vi "VIQueryBuildSpecs.vi"(8 "Error In":errorcluster, 11 "Project Path":string) -> (0 "Error Out":errorcluster, 3 "Targets":T1[](array[typedef]))   [LabVIEW 2013]
uses:
  VIProject/VPTargetBuildSpecs.ctl
  VIProject/VPBuildSpecInformation.ctl
  VIProject/VIProject.lvlib
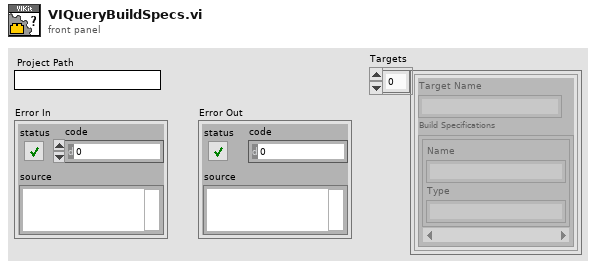
[diagram p1: front panel]
types:
  T1 = typedef "VIProject.lvlib/VPTargetBuildSpecs.ctl" = cluster{"Target Name":string, "Build Specifications":T2[]}
  T2 = typedef "VIProject.lvlib/VPBuildSpecInformation.ctl" = cluster{"Name":string, "Type":string}
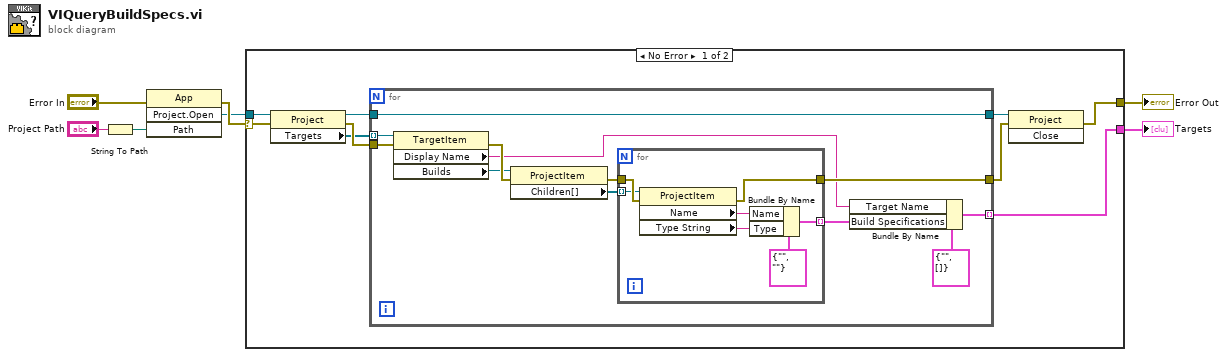
[diagram p0: block diagram]
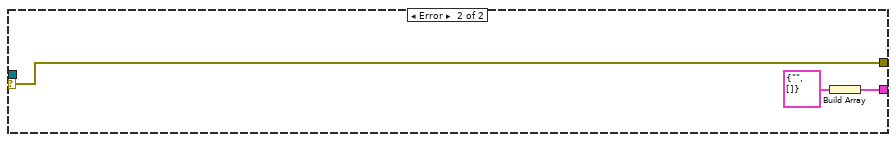
[diagram p2: hidden frame]
diagram:
  n1 = String To Path(string="Project Path") -> (path=w2:path)
  n2 = invoke class="App" method="Project.Open"(error in="Error In", "Path"=w2) -> (error out=w5:errorcluster, "Project:Open"=w4:refnum<vi>)  [unwired: 2 in, 2 out]
  n3 = case shown="No Error" w5 {
    selector: w5 -> [w9 w38]
    tunnel: [w14 w36] -> w7
    tunnel: [w10 w38] -> w6
    tunnel: w4 -> [w8 _]
    frame No Error {
      n4 = property class="Project"(reference=w8, error in=w9) -> (reference out=w13:refnum<vi>, error out=w16:errorcluster, "Targets"=w15:refnum<vi>[])
      n5 = for {
        tunnel: w15 -> [w28] mode=indexing
        tunnel: w16 -> [w27]
        tunnel: [w23] -> w14 mode=indexing
        tunnel: [w22] -> w11
        tunnel: [w17] -> w12
        tunnel: w13 -> [w17]
        n6 = property class="TargetItem"(reference=w28, error in=w27) -> (error out=w26:errorcluster, "Display Name"=w21:string, "Builds"=w18:refnum<vi>)  [unwired: 1 out]
        n7 = property class="ProjectItem"(reference=w18, error in=w26) -> (error out=w25:errorcluster, "Children[]"=w24:refnum<vi>[])  [unwired: 1 out]
        n8 = for {
          tunnel: w25 -> [w34]
          tunnel: w24 -> [w33] mode=indexing
          tunnel: [w35] -> w22
          tunnel: [w30] -> w19 mode=indexing
          n9 = property class="ProjectItem"(reference=w33, error in=w34) -> (error out=w35:errorcluster, "Name"=w32:string, "Type String"=w31:string)  [unwired: 1 out]
          n10 = Bundle By Name(cluster=T2 {"Name"="", "Type"=""} ("Build Specification Information"), "Name"=w32, "Type"=w31) -> (w30:T2)
        }
        n11 = Bundle By Name(cluster=T1 {"Target Name"="", "Build Specifications"=[]} ("Build Specification"), "Target Name"=w21, "Build Specifications"=w19) -> (w23:T1)
      }
      n12 = invoke class="Project" method="Close"(reference=w12, error in=w11) -> (error out=w10:errorcluster)  [unwired: 1 in, 2 out]
    }
    frame Error {
      n13 = Build Array(T1 {"Target Name"="", "Build Specifications"=[]} ("Build Specification")) -> (w36:T1[])
    }
  }
  "Error Out" <- w6
  "Targets" <- w7
